vi "Dashboard Main.vi"() -> ()   [LabVIEW 2015]
uses:
  <vilib>/Utility/miscctls.llb/LVRowAndColumnTypeDef.ctl
  <vilib>/event_ctls.llb/eventvkey.ctl
  <vilib>/Rock Robotics/WPI/Dashboard/WPI_DashboardLogging Global.vi
  <vilib>/Rock Robotics/Network Tables/NT Read Numeric Array.vi
  <vilib>/Rock Robotics/Network Tables/NT Read Boolean.vi
  <vilib>/Rock Robotics/Network Tables/NT Write Boolean.vi
  <vilib>/functionblocks/Edge Detection/One Shot Rising with Input/One Shot Rising with Input.vi
  <vilib>/Utility/config.llb/Write Key (String).vi
  <vilib>/Utility/config.llb/Write Key (I32).vi
  <vilib>/functionblocks/FB Core/FB Core.xnode
  <vilib>/Utility/config.llb/NI_LVConfig.lvlib
  <vilib>/functionblocks/NI_FunctionBlock Libraries.lvlib
panel:
  in  "TCP":refnum<k5>
  in  "Rec Mode":enum32{"Stop", "Record", "Playback"}(radio)
  in  "Vision":u16(ring) items=["Camera Off", "USB Camera SW", "USB Camera HW", "IP Camera"]
  out "Camera IP":string
  out "Image Message":string="Timeout in Camera Communications"
  in  "Dashboard Tab":T1(tab)
  in  "Select Auto":string(combo)
  out "NT Connection":bool
  in  "Camera Settings":T2={"Frame Rate"=30, "Compression"=30, "Size"=1} {"Frame Rate" scale=1.0..30.0; "Size" items=["640x480", "320x240", "160x120"]}
  out "MotorChart R":cluster{"Numeric":dbl, "Numeric":dbl}(graph)
  out "MotorChart L":T3(graph)
  out "MotorSliders R":cluster{"MotorSlide1":dbl, "MotorSlide2":dbl} {"MotorSlide2" scale=-1.0..1.0 scale format="%#_2e"; "MotorSlide1" scale=-1.0..1.0 scale format="%#_2e"}
  out "MotorSliders L":T4 {"MotorSlide4 2" scale=0.0..14.0 scale format="%#_2e"; "MotorSlide2" scale=-1.0..1.0 scale format="%#_2e"; "MotorSlide1" scale=-1.0..1.0 scale format="%#_2e"}
  out "Gyro":dbl(knob) scale=0.0..360.0
  out "JS1 Z":dbl(slide) scale=-1.0..1.0 scale format="%#_2e"
  out "JS1 Graph":cluster{"X":dbl, "Y":dbl}[](graph)
  out "JS1 Buttons":T5
  out "JS2 Z":dbl(slide) scale=-1.0..1.0 scale format="%#_2e"
  out "JS2 Graph":cluster{"X":dbl, "Y":dbl}[](graph)
  out "JS2 Buttons":T5
  out "Mode":T6(ring)=enum."Auto Disabled"
  in  "DB Camera Config":bool
  out "fps":dbl format="%#.1g"
  out "Mbps":dbl format="%#.1g"
  out "Mbps LED":bool
  out "Image Out":T7(plugin-control)
  out "Drawing Box":bool
  in  "Auto Mode":enum16{"No Auto", "Simple Auto", "Shoot Auto"}(ring)
  in  "Push Camera Values":bool
  in  "Sat Min":dbl
  in  "Sat Max":dbl
  in  "Val Min":dbl
  in  "Val Max":dbl
  in  "Hue Min":dbl
  in  "Hue Max":dbl
  in  "Camera calibration":bool
  out "SHOOTER FAULT":bool
  out "Mode":string
  out "Shooter":dbl(slide) scale=0.0..80000.0
  out "Tilt":dbl(slide) scale=0.0..750.0
  out "Elevation":dbl(slide) scale=0.0..45000.0
  out "ELEVATOR FAULT":bool
  out "TILT FAULT":bool
  in  "Test Slider":dbl(slide) scale=0.0..100.0 scale format="%#_3g"
  in  "On/Off":bool caption="Solenoid"
  in  "Test Name":u16(ring) items=["Select the test to run..."]
  in  "Test Tree":string(tree)
  in  "Motor":cluster{"Value":dbl, "Enable":bool} {"Value" scale=-1.0..1.0 scale format="%#_3g"}
  out "Progress":T8 {"Test Progress" scale=0.0..100.0}
  in  "Rev/Fwd":cluster{"Forward":bool, "Reverse":bool}
  in  "Test Ring":u16(ring) items=["Monochrome", "Color"]
  out "Cmd Status":string
  in  "Execute Command":bool
  in  "Command Params":string[][](table)
  in  "Command Selection":i32(listbox)
  in  "CheckList":i32(listbox)
  out "Tree":string(tree)
  out "Camera Image":T7(plugin-control)
  out "Background":bool
  # "Left"
  # "Front"
  # "Right"
  # "Battery"
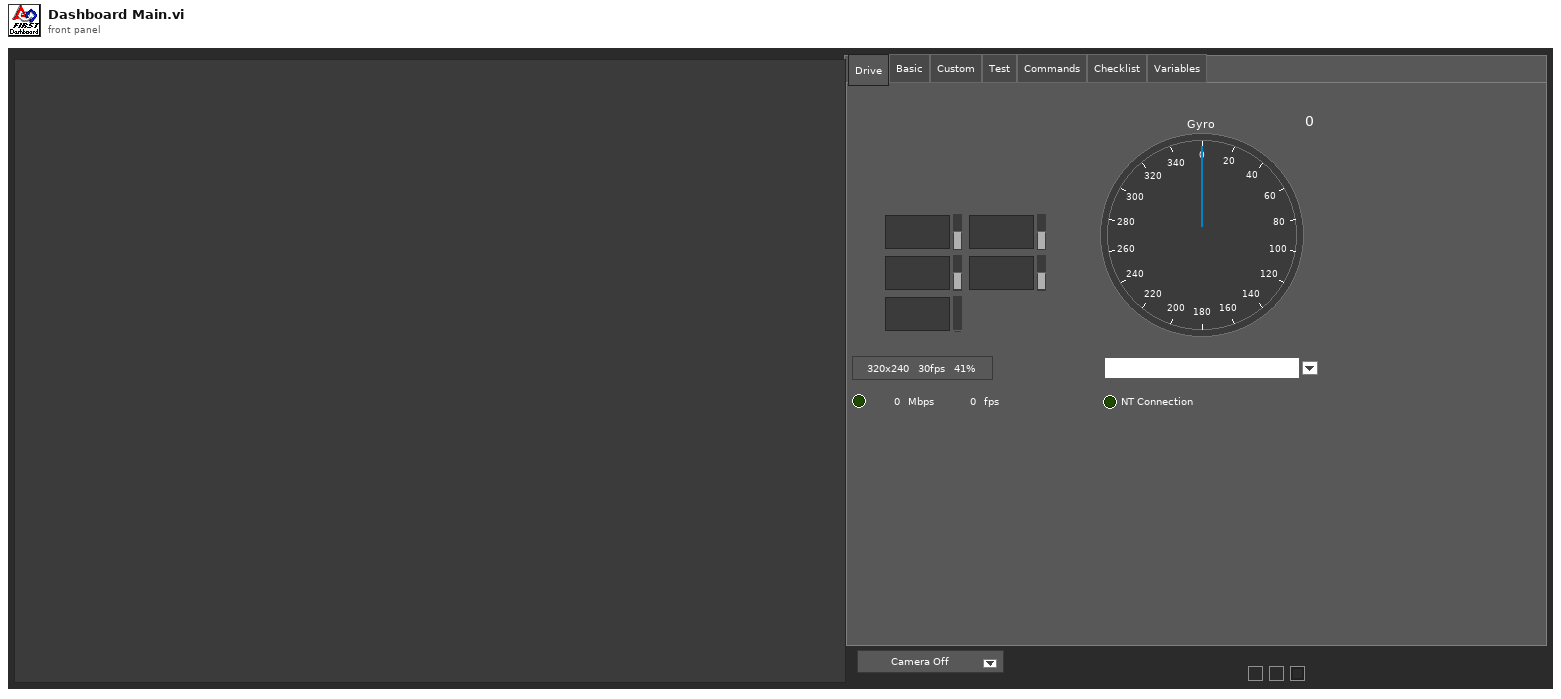
[diagram p1: front panel]
types:
  T1 = enum32{"Drive", "Basic", "Custom", "Test", "Commands", "Checklist", "Variables"}
  T2 = cluster{"Frame Rate":i32, "Compression":i32, "Size":u16}
  T3 = cluster{"Numeric":dbl, "Numeric":dbl, "Battery V":dbl}
  T4 = cluster{"MotorSlide1":dbl, "MotorSlide2":dbl, "MotorSlide4 2":dbl}
  T5 = cluster{bool, bool, bool, bool, bool, bool, bool, bool, bool, bool, bool, bool}
  T6 = enum8{"Tele-Op Disabled", "Tele-Op Enabled", "Auto Disabled", "Auto Enabled", "Test Disabled", "Test Enabled", "Disconnected", "No Code", "E-Stop"}
  T7 = typedef "IMAQ Image.ctl" = refnum<image>
  T8 = cluster{"Test Progress":u8, "Test Progress Text":string}
  T9 = cluster{"IDs":cluster{"RPC field ID":u16, "Unique ID":u16}, "String":string}
  T10 = enum32{"Drive", "Basic", "Custom", "Test", "Checklist", "Variables"}
  T11 = typedef "Image Type" = u32
  T12 = cluster{"Camera Image":refnum<vi>, "Dashboard Tab":refnum<vi>, "Background":refnum<vi>, "Vision":refnum<vi>, "Rec Mode":refnum<vi>, "Test Slider":refnum<vi>, "On/Off ":refnum<vi>, "Test Ring":refnum<vi>, "Rev/Fwd":refnum<vi>, "Test Name":refnum<vi>, "Motor":refnum<vi>, "Progress":refnum<vi>, "CheckList":refnum<vi>, "Tree":refnum<vi>, "Test Tree":refnum<vi>, "Command Params":refnum<vi>, "Command Selection":refnum<vi>, "Execute Command":refnum<vi>, "Cmd Status":refnum<vi>}
  T13 = cluster{"Error Strings":string, "Disable Counts":cluster{u16, u16}, "Rail Faults":cluster{u16, u16, u16}, "Robot IP":string, "DB Mode":u8, "Event Info":cluster{"Name":string, "Type":u8, "Number":u16, "Replay":u8}, "Camera Addr":string}
  T14 = cluster{"Storage":cluster{"Disk Free":u64, "RAM Block":u32, "RAM free":u32}, "CPU Utilization":cluster{"CPU % ISR":sgl, "CPU % Time Crit":sgl, "CPU % Timed Str":sgl, "CPU % High":sgl, "CPU % Above":sgl, "CPU % Normal":sgl, "CPU % Low":sgl}, "CAN":cluster{"% Bus Utilization":sgl, "Bus Off Cnt":u32, "TX_FIFO Full Cnt":u32, "Receive Error Cnt":u8, "Transmit Error Cnt":u8}, "HID":cluster{"HID Outputs":u32, "Rumble Low":u16, "Rumble High":u16}[]}
  T15 = cluster{"Status bits":cluster{"Test Mode":bool, "Autonomous":bool, "Enabled":bool, "Code Start":bool, "Brownout":bool, "Reserved 2":bool, "Reserved 3":bool, "E-Stop":bool}, "Code Trace":cluster{"Disabled":bool, "TeleOp":bool, "Auto":bool, "Test":bool}, "Controller Type":enum16{"unknown", "cRIO", "roboRio"}, "Code?":enum16{"unknown", "noCode", "code"}, "Battery V":dbl}
  T16 = cluster{"Control Bits":cluster{"TestMode":bool, "Autonomous":bool, "Enabled":bool, "FMS Present":bool, bool, bool, bool, "E-Stop":bool}, "Team Station ":u8, "Countdown":sgl, "Joystick Values":cluster{"Axes":dbl[], "Buttons":bool[], "POVs":i16[]}[]}
  T17 = cluster{"Axes":dbl[], "Buttons":bool[], "POVs":i16[]}[]
  T18 = cluster{"Axes":dbl[], "Buttons":bool[], "POVs":i16[]}
  T19 = cluster{"Buttons[0]":bool, "Buttons[1]":bool, "Buttons[2]":bool, "Buttons[3]":bool, "Buttons[4]":bool, "Buttons[5]":bool, "Buttons[6]":bool, "Buttons[7]":bool, "Buttons[8]":bool, "Buttons[9]":bool, "Buttons[10]":bool, "Buttons[11]":bool}
  T20 = typedef "NI_LVConfig.lvlib/Config Data RefNum.ctl" = refnum<k1>
  T21 = cluster{"Operation":enum16{"Update", "Clear"}, "Color Box":u32}[]
  T22 = typedef "eventvkey.ctl" = enum16{"ASCII", "Enter", "Return", "Shift", "Ctrl", "Alt", "Cmd", "Opt", "Caps", "NumLock", "Clear", "Break", "Up", "Down", "Left", "Right", "Insert", "Delete", "Home", "End", "PageUp", "PageDown", "Escape", "Help", "Pause", "ScrollLock", "F1", "F2", "F3", "F4", "F5", "F6", "F7", "F8", "F9", "F10", "F11", "F12", "F13", "F14", "F15", "F16", "F17", "F18", "F19", "F20", "F21", "F22", "F23", "F24", "Play", "VolumeUp", "VolumeDown", "Mute", "Two Byte Char"}
  T23 = cluster{"Image Size":bool, "Image Type":bool, "Pixel Value":bool, "ROI Information":bool, "Zoom Factor":bool}
  T24 = enum8{"Enabled", "Disabled", "Disabled and Grayed Out"}
  T25 = cluster{"Operation":enum16{"Update", "Clear"}, "Color Box":u32}
  T26 = typedef "LVRowAndColumnTypeDef.ctl" = cluster{"Row":i32, "Column":i32}
  T27 = cluster{"Shift":bool, "Ctrl":bool, "Alt":bool, "Cmd":bool, "Opt":bool}
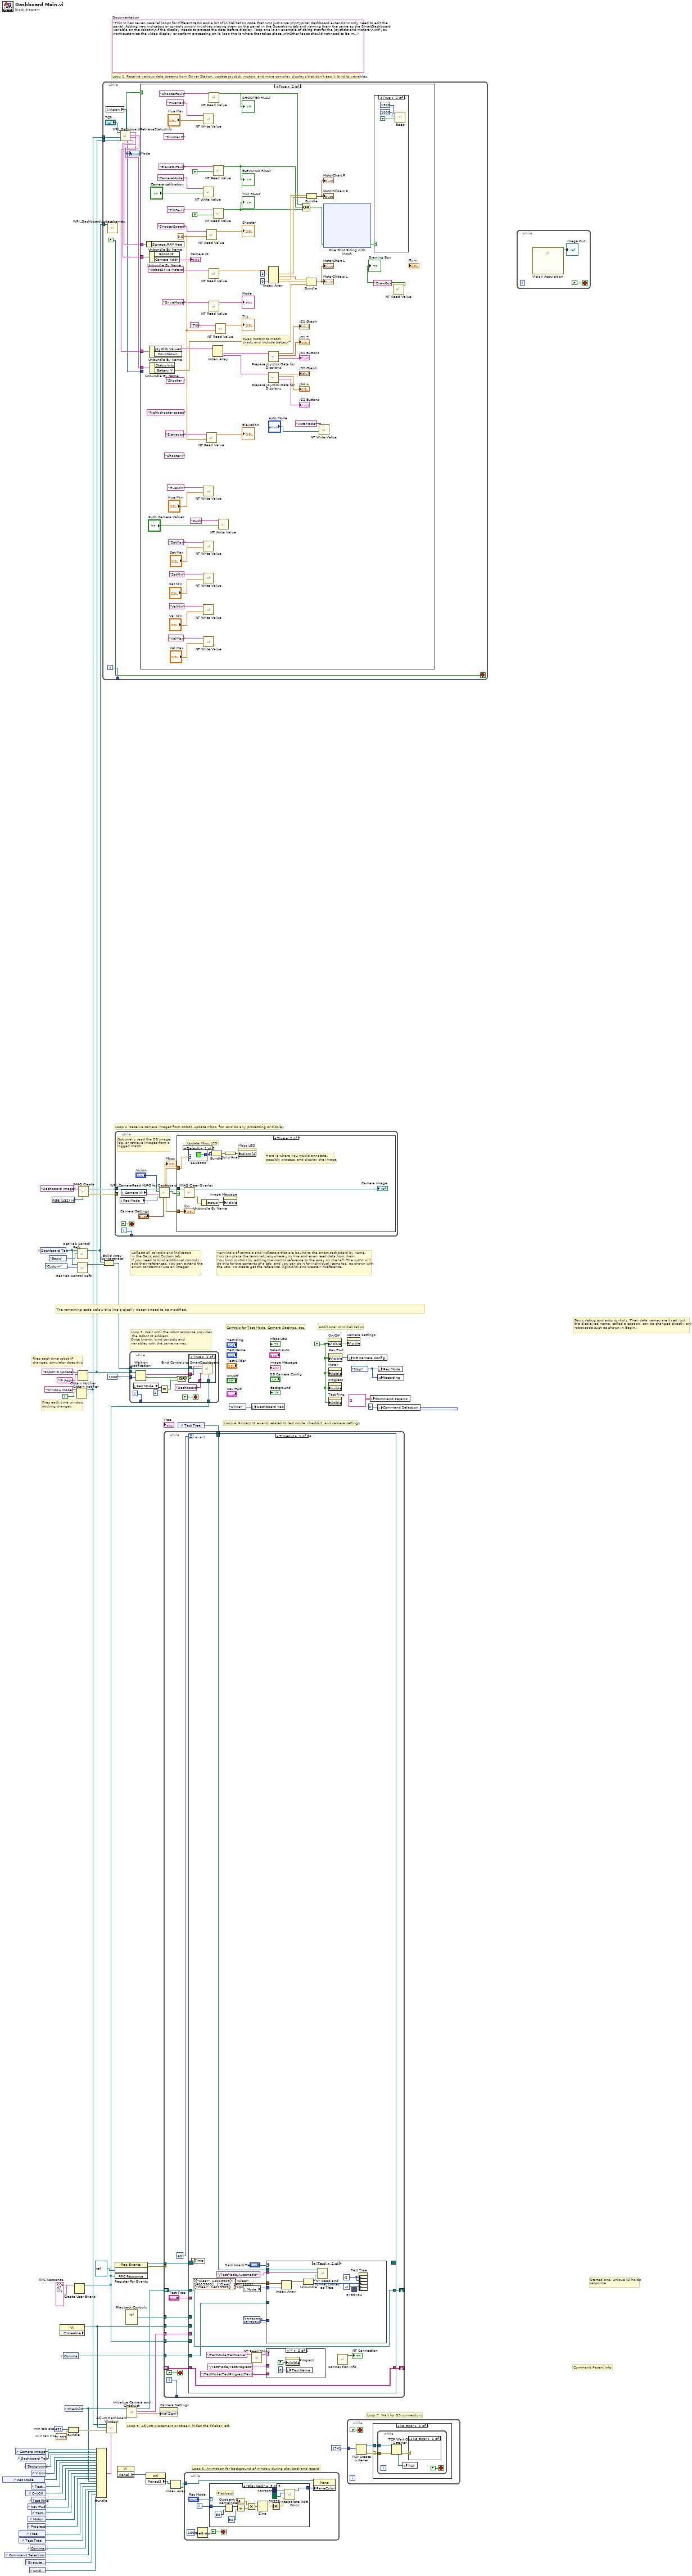
[diagram p0: block diagram]
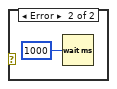
[diagram p2: hidden frame]
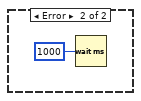
[diagram p3: hidden frame]
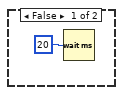
[diagram p4: hidden frame]
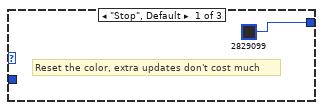
[diagram p6: hidden frame]
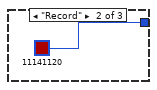
[diagram p7: hidden frame]
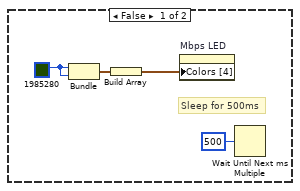
[diagram p9: hidden frame]
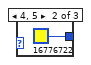
[diagram p10: hidden frame]
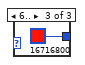
[diagram p11: hidden frame]
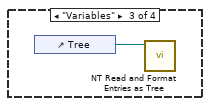
[diagram p13: hidden frame]
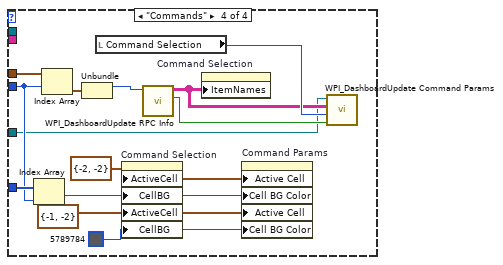
[diagram p14: hidden frame]
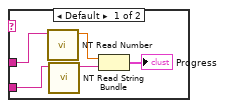
[diagram p15: hidden frame]
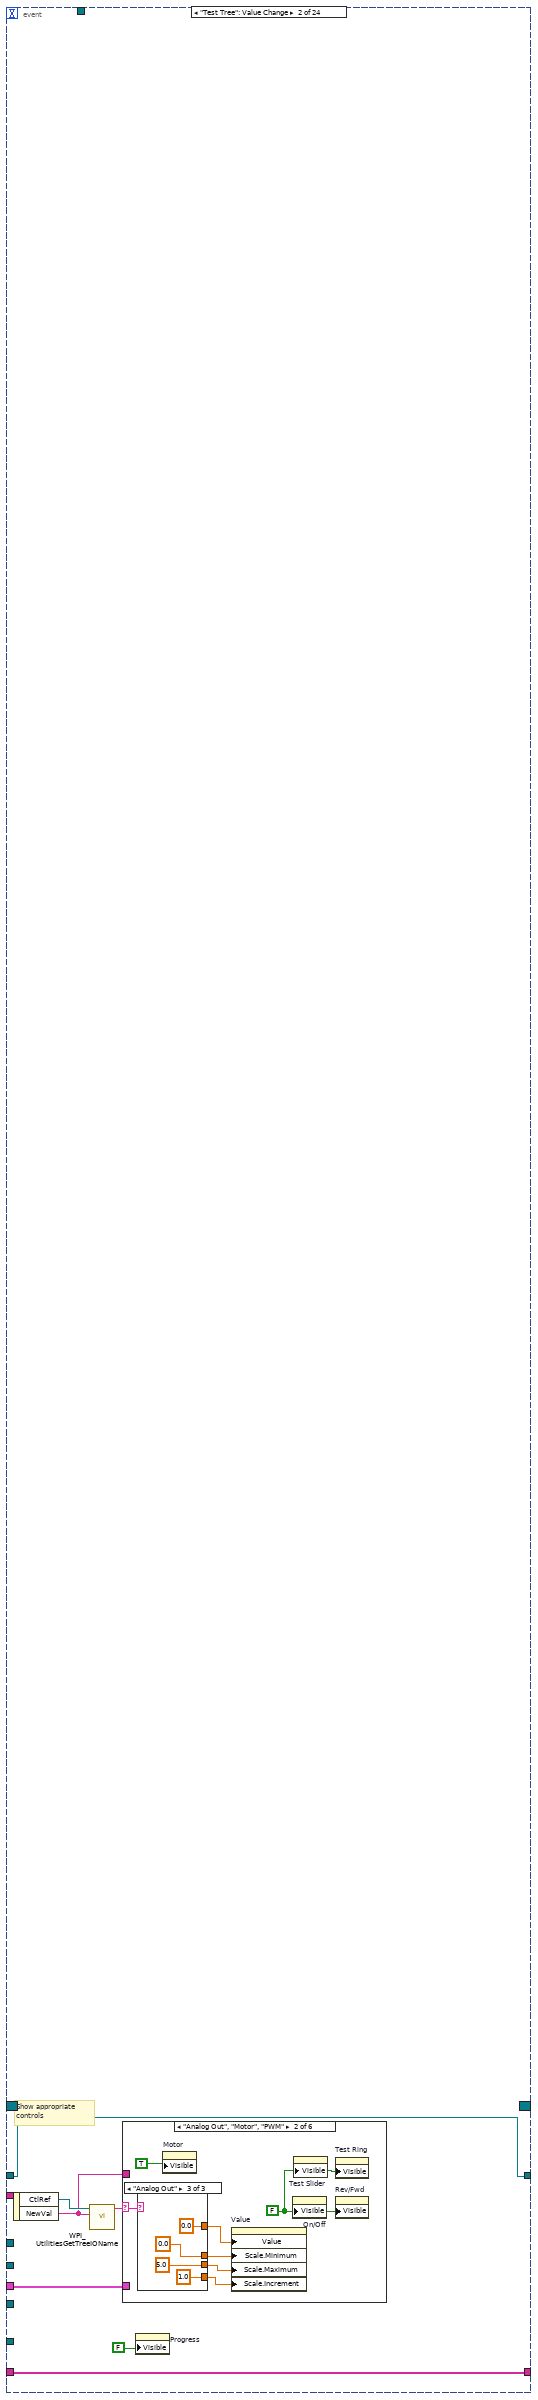
[diagram p16: hidden frame]
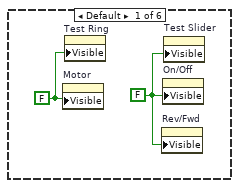
[diagram p17: hidden frame]
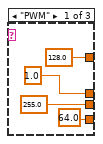
[diagram p18: hidden frame]
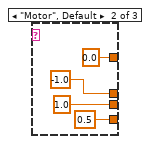
[diagram p19: hidden frame]
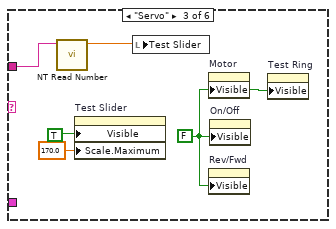
[diagram p20: hidden frame]
diagram:
  w7 = T9 {"IDs"={"RPC field ID"=0, "Unique ID"=0}, "String"=""}  # RPC Response
  w33 = 491  # min tab size
  w32 = 1.333  # min tab size
  w41 = enum32{"Stop", "Record", "Playback"}."Stop" ("Rec Mode")
  w15 = FALSE ("Visible")
  (unwired) "This VI has seven parallel loops for different tasks and a bit of initialization code that runs just once.\n\nTypical dashboard extensions only need to edit the panel. Adding new indicators or controls simply involves placing them on the panel in the Operations tab and naming them the same as the SmartDashboard variable on the robot\n\nIf the display needs to process the data before display, loop one is an example of doing that for the joysticks and motors.\n\nIf you want customize the video display or perform processing on it, loop two is where that takes place.\n\nOther loops should not need to be modified. They are pretty standard, and document the task they perform."  # Documentation
  w61 = T11 4 items=["Grayscale (U8)", "Grayscale (I16)", "Grayscale (SGL)", "Complex (CSG)", "RGB (U32)", "HSL (U32)", "RGB (U64)"] ("Image Type")
  # "Command Param Info"
  # "Started one, Unique ID holds\nresponse"
  # "Loop 7. Wait for DS connections"
  # "Basic debug and auto controls: Their data names are fixed, but\nthe displayed name, called a caption, can be changed directly or in\nrobot code such as shown in Begin."
  # "Controls for Test Mode, Camera Settings, etc."
  # "Additional UI Initialization"
  # "Loop 6. Animation for background of window during playback and record"
  # "Fires each time robot IP\nchanges, simulator does this"
  # "Fires each time window\ndocking changes."
  # "Collects all controls and indicators\nin the Basic and Custom tab.\nIf you need to bind additional controls,\nadd their references. You can extend the\nenum constant or use an integer."
  # "The remaining code below this line typically doesn't need to be modified."
  # "Loop 4. Process UI events related to test mode, checklist, and camera settings"
  # "Terminals of controls and indicators that are bound to the smart dashboard by name.\nYou can place the terminals anywhere you like and even read data from them.\nYou bind controls by adding the control reference to the array on the left. The subVI will\ndo this for the contents of a tab, and you can do it for individual items too, as shown with\nthe LED. To create get the reference, right-click and Create>>Reference."
  # "Loop 3. Wait until the robot response provides\n the Robot IP address.\nOnce known, bind controls and\nvariables with the same names."
  # "Loop 5. Adjusts placement onscreen, hides the titlebar, etc."
  # "Loop 1. Receive various data streams from Driver Station, update joystick, motors, and more complex displays that don't easily bind to variables."
  # "Loop 2. Receive camera images from Robot, update Mbps, fps, and do any processing or display"
  n1 = control-ref of="Rec Mode"() -> (w21:refnum<vi>)
  n2 = control-ref of="Command Selection"() -> (w6:refnum<vi>)
  n3 = control-ref of="Camera Image"() -> (w36:refnum<vi>)
  n4 = control-ref of="Tree"() -> (w25:refnum<vi>)
  n5 = control-ref of="Test Tree"() -> (w24:refnum<vi>)
  n6 = control-ref of="Dashboard Tab"() -> (w35:refnum<vi>)
  n7 = control-ref of="Execute Command"() -> (w8:refnum<vi>)
  n8 = control-ref of="Background"() -> (w30:refnum<vi>)
  n9 = control-ref of="On/Off"() -> (w19:refnum<vi>)
  n10 = control-ref of="Progress"() -> (w16:refnum<vi>)
  n11 = control-ref of="Rev/Fwd"() -> (w17:refnum<vi>)
  n12 = control-ref of="Motor"() -> (w22:refnum<vi>)
  n13 = control-ref of="Cmd Status"() -> (w2:refnum<vi>)
  n14 = control-ref of="Command Params"() -> (w9:refnum<vi>)
  n15 = control-ref of="Test Slider"() -> (w20:refnum<vi>)
  n16 = control-ref of="Vision"() -> (w34:refnum<vi>)
  n17 = control-ref of="Test Ring"() -> (w18:refnum<vi>)
  n18 = control-ref of="Test Name"() -> (w23:refnum<vi>)
  n19 = control-ref of="Dashboard Tab"() -> (w39:refnum<vi>)
  n20 = property class="VI" props=["Front Panel.Closeable"]() -> (reference out=w40:refnum<vi>)  [unwired: 2 in, 2 out]
  n21 = control-ref of="Command Params"() -> (w1:refnum<vi>)
  n22 = control-ref of="CheckList"() -> (w26:refnum<vi>)
  n23 = Bundle("min tab size"=w33, "min tab size"=w32) -> (w31:cluster{"min tab size":i32, "min tab size":dbl})  [unwired: 1 in]
  n24 = Create User Event(user event datatype=w7) -> (user event=w3:refnum<user-event>)  [unwired: 1 in, 1 out]
  n25 = Obtain Notifier(name (unnamed)="Window Mode", notification data type=TRUE) -> (notifier out=w12:refnum<notifier>)  [unwired: 2 in, 2 out]
  n26 = call <vilib>:"Get Tab Control Refs.vi"("Page Index"=T10."Basic" ("Dashboard Tab"), "TabControl in"=w39) -> ("ControlsOnPage"=w13:refnum<vi>[])  [unwired: 9 in]
  n27 = call <vilib>:"Get Tab Control Refs.vi"("Page Index"=T10."Custom" ("Dashboard Tab"), "TabControl in"=w39) -> ("ControlsOnPage"=w38:refnum<vi>[])  [unwired: 9 in]
  n28 = Obtain Notifier(name (unnamed)="Robot IP Update", notification data type="IP Addr" ("name (unnamed)")) -> (notifier out=w14:refnum<notifier>)  [unwired: 2 in, 2 out]
  n29 = call "IMAQ Create"("Image Name"="Dashboard Image", "Image Type"=w61) -> ("New Image"=w59:T7, "error out"=w58:errorcluster)  [unwired: 2 in, 1 out]
  n30 = Bundle("Camera Image"=w36, "Dashboard Tab"=w35, "Background"=w30, "Vision"=w34, "Rec Mode"=w21, "Test Slider"=w20, "On/Off"=w19, "Test Ring"=w18, "Rev/Fwd"=w17, "Test Name"=w23, "Motor"=w22, "Progress"=w16, "CheckList"=w26, "Tree"=w25, "Test Tree"=w24, "Command Params"=w9, "Command Selection"=w6, "Execute Command"=w8, "Cmd Status"=w2) -> (w27:T12)  [unwired: 1 in]
  n31 = while {
    tunnel: [w73] -> _
    tunnel: w14 -> [w67]
    tunnel: w13 -> [w66]
    tunnel: w12 -> [w62]
    i -> [w73]
    stop <- FALSE stop-if-true
    n32 = local read "Vision"() -> (w64:u16)
    n33 = call <vilib>:"WPI_DashboardUpdateNames.vi"("Controls on Tab"=w66) -> ()  [unwired: 11 in]
    n34 = call <vilib>:"WPI_DashboardRetrieveStatusInfo.vi"("Vision"=w64, "Binding Refnum"=w67, "Window Mode Notifier"=w62, "TCP Cnx"="TCP") -> ("Power and Errors"=w68:T13, "Robot Metrics"=w71:T14, "Status Info"=w72:T15, "Control Info"=w69:T16, "Robot Mode"=w65:T6, "Process?"=w70:bool)  [unwired: 2 in]
    "Mode" <- w65
    n35 = case shown="True" w70 {
      tunnel: w72 -> [_ w139]
      tunnel: w71 -> [_ w138]
      tunnel: w69 -> [_ w137]
      tunnel: w68 -> [_ w136]
      tunnel: w65 -> [_ _]
      frame False {
        n36 = Wait (ms)(milliseconds to wait=u32 20) -> ()  [unwired: 1 out]
      }
      frame True {
        (unwired) "Shooter D" ("Name")
        (unwired) "Shooter I" ("Name")
        (unwired) "Shooter P" ("Name")
        (unwired) "Right shooter speed" ("Name")
        w105 = 0.0 ("Default Value")
        # "swap motors to match\ncharts and include battery"
        n37 = Unbundle By Name(w138) -> ()  [unwired: 1 out]
        n38 = Unbundle By Name(w137) -> ("Joystick Values"=w126:T17)  [unwired: 1 out]
        n39 = Unbundle By Name(w136) -> ("Camera Addr"=→"Camera IP":string)  [unwired: 1 out]
        n40 = Unbundle By Name(w139) -> ("Battery V"=w127:dbl)  [unwired: 1 out]
        n41 = call-poly <vilib>:"NT Write Value.vi"("Boolean"="Camera calibration", "Name"="CameraMode") -> ()  [unwired: 9 in, 1 out]
        n42 = call-poly <vilib>:"NT Write Value.vi"("Numeric"="Hue Max", "Name"="HueMax") -> ()  [unwired: 9 in, 1 out]
        n43 = call-poly <vilib>:"NT Write Value.vi"("Numeric"="Hue Min", "Name"="HueMin") -> ()  [unwired: 9 in, 1 out]
        n44 = call-poly <vilib>:"NT Write Value.vi"("Numeric"="Sat Max", "Name"="SatMax") -> ()  [unwired: 9 in, 1 out]
        n45 = call-poly <vilib>:"NT Write Value.vi"("Numeric"="Sat Min", "Name"="SatMin") -> ()  [unwired: 9 in, 1 out]
        n46 = call-poly <vilib>:"NT Write Value.vi"("Numeric"="Val Min", "Name"="ValMin") -> ()  [unwired: 9 in, 1 out]
        n47 = call-poly <vilib>:"NT Write Value.vi"("Numeric"="Val Max", "Name"="ValMax") -> ()  [unwired: 9 in, 1 out]
        n48 = call-poly <vilib>:"NT Read Value.vi"("Default Value"=w105, "Name"="ShooterSpeed") -> ("Numeric"=→"Shooter":dbl)  [unwired: 8 in, 1 out]
        n49 = call-poly <vilib>:"NT Read Value.vi"("Default Value"=w105, "Name"="Elevation") -> ("Numeric"=→"Elevation":dbl)  [unwired: 8 in, 1 out]
        n50 = call-poly <vilib>:"NT Read Value.vi"("Name"="ShooterFault") -> ("Boolean"=w100:bool)  [unwired: 9 in, 1 out]
        "SHOOTER FAULT" <- w100
        n51 = call-poly <vilib>:"NT Read Value.vi"("Name"="RobotDrive Motors") -> ("Numeric Array"=w115:dbl[])  [unwired: 9 in, 1 out]
        n52 = call-poly <vilib>:"NT Read Value.vi"("Name"="DriveMode") -> ("String"=→"Mode":string)  [unwired: 9 in, 1 out]
        n53 = Index Array(array=w126) -> (element #1=w125:T18, element #2=w120:T18)  [unwired: 2 in]
        n54 = call-poly <vilib>:"NT Read Value.vi"("Default Value"=FALSE, "Name"="ElevatorFault") -> ("Boolean"=w101:bool)  [unwired: 8 in, 1 out]
        "ELEVATOR FAULT" <- w101
        n55 = call-poly <vilib>:"NT Read Value.vi"("Default Value"=FALSE, "Name"="TiltFault") -> ("Boolean"=w99:bool)  [unwired: 8 in, 1 out]
        "TILT FAULT" <- w99
        n56 = call-poly <vilib>:"NT Read Value.vi"("Default Value"=w105, "Name"="Tilt") -> ("Numeric"=→"Tilt":dbl)  [unwired: 8 in, 1 out]
        n57 = call-poly <vilib>:"NT Write Value.vi"("Boolean"="Push Camera Values", "Name"="Push") -> ()  [unwired: 9 in, 1 out]
        n58 = Index Array(array=w115, index #1=1, index #4=0) -> (element #1=w131:dbl, element #2=w132:dbl, element #3=w130:dbl, element #4=w135:dbl)  [unwired: 2 in]
        n59 = call "Prepare Joystick Data for Displays.vi"("Joystick Values"=w125) -> ("Buttons"=→"JS1 Buttons":T19, "Z Axis"=→"JS1 Z":dbl, "Cartesian Data"=→"JS1 Graph":cluster{"X axis":dbl, "X axis":dbl}[])  [unwired: 8 in]
        n60 = call "Prepare Joystick Data for Displays.vi"("Joystick Values"=w120) -> ("Buttons"=→"JS2 Buttons":T19, "Z Axis"=→"JS2 Z":dbl, "Cartesian Data"=→"JS2 Graph":cluster{"X axis":dbl, "X axis":dbl}[])  [unwired: 8 in]
        n61 = Compound Arithmetic op=OR(w100, w101, w99) -> (w98:bool)
        n62 = Bundle("Numeric"=w132, "Numeric"=w135, "Battery V"=w127) -> (→"MotorChart L" →"MotorSliders L":T3)  [unwired: 1 in]
        n63 = Bundle("Numeric"=w130, "Numeric"=w131) -> (→"MotorChart R" →"MotorSliders R":cluster{"Numeric":dbl, "Numeric":dbl})  [unwired: 1 in]
        n64 = call-poly <vilib>:"NT Write Value.vi"("Numeric"="Auto Mode", "Name"="AutoMode") -> ()  [unwired: 9 in, 1 out]
        n65 = xnode "One Shot Rising with Input"("input"=w98) -> ("output"=w97:bool)  [unwired: 1 in, 1 out]
        n66 = case shown="True" w97 {
          frame False {
          }
          frame True {
            n67 = call <vilib>:"Beep.vi"("use system alert? (T)"=FALSE, "duration (msec)"=u32 1000, "frequency (Hz)"=u32 1500) -> ()  [unwired: 9 in]
          }
        }
        n68 = call-poly <vilib>:"NT Read Value.vi"("Name"="DrawBox") -> ("Boolean"=→"Drawing Box":bool)  [unwired: 9 in, 1 out]
      }
    }
  }
  n69 = Build Array (concatenate)(w13, w38) -> (w37:refnum<vi>[])
  n70 = call "Adjust Dashboard Window.vi"("Sizing Refnums"=w27, "Size Constraints"=w31, "VI"=w40, "WIn Mode"=w12) -> ()  [unwired: 8 in]
  n71 = while {
    tunnel: w59 -> [w189]
    tunnel: w58 -> [_]
    tunnel: [w190] -> _
    i -> [w190]
    stop <- FALSE stop-if-true
    # "Optionally read the DB image,\nlog, or retrieve images from a\nlogged match"
    n72 = local read "Rec Mode"() -> (w184:enum32{"Stop", "Record", "Playback"})
    n73 = local read "Camera IP"() -> (w182:string)
    n74 = call <vilib>:"WPI_CameraRead MJPG for Dashboard.vi"("Camera Settings"="Camera Settings", "Rec Mode"=w184, "Camera IP"=w182, "Camera Mode"="Vision", "Refnum in"=w189) -> ("Active"=w187:bool, "Refnum out"=w188:T7, "FPS"=w186:dbl, "Bandwidth (Mbps)"=w181:dbl)  [unwired: 3 in]
    "Mbps" <- w181
    n75 = case shown="True" w187 {
      tunnel: w188 -> [_ w199]
      tunnel: w181 -> [_ w198]
      tunnel: w186 -> [_ w196]
      frame False {
        w192 = u32 1985280 ("Color Box")
        # "Sleep for 500ms"
        n76 = Bundle("Color Box"=w192, "Color Box"=w192) -> (w194:cluster{"Color Box":u32, "Color Box":u32})  [unwired: 1 out]
        n77 = Build Array(w194) -> (w193:cluster{"Color Box":u32, "Color Box":u32}[])
        n78 = property on="Mbps LED" class="Bool (strict)"("Colors [4]"=w193) -> ()  [unwired: 2 in, 2 out]
        n79 = Wait Until Next ms Multiple(millisecond multiple=u32 500) -> ()  [unwired: 1 out]
      }
      frame True {
        # "Here is where you would annotate,\npossibly process, and display the image"
        # "Update Mbps LED"
        n80 = call "IMAQ Clear Overlay"("Image"=w199) -> ("error out"=w203:errorcluster, "Image Out"=→"Camera Image":T7)  [unwired: 2 in, 7 out]
        n81 = case shown="Default" w198 {
          tunnel: [u32 6618880 ("Color Box") u32 16776722 ("Color Box") u32 16716800 ("Color Box")] -> w200
          frame Default {
          }
          frame 4, 5 {
          }
          frame 6.. {
          }
        }
        n82 = Unbundle By Name(w203) -> ("status"=w204:bool)
        n83 = Bundle("Color Box"=w200, "Color Box"=w200) -> (w202:cluster{"Color Box":u32, "Color Box":u32})  [unwired: 1 out]
        n84 = property on="Image Message" class="Str"("Visible"=w204) -> ()  [unwired: 2 in, 2 out]
        n85 = Build Array(w202) -> (w201:cluster{"Color Box":u32, "Color Box":u32}[])
        n86 = property on="Mbps LED" class="Bool (strict)"("Colors [4]"=w201) -> ()  [unwired: 2 in, 2 out]
        "fps" <- w196
      }
    }
  }
  n87 = register-events(refnum<vi> refnum, w3) -> (reference out=w45:refnum<event-registration>, error out=w44:errorcluster)  [unwired: 2 in]
  n88 = property class="VI"() -> ("Panel"=w48:refnum<vi>)  [unwired: 2 in, 2 out]
  n89 = vi-ref "Playback Controls.vi"() -> (w46:refnum<vi>)
  n90 = call "Initialize Camera and CheckList.vi"("ListBox in"=w26) -> ("Cluster"=w52:cluster{"value":i32, "value":i32, "index":i32}, "Array"=w53:cluster{string[]}[], "File Refnum"=w51:T20)  [unwired: 8 in]
  n91 = while {
    tunnel: w37 -> [w220]
    tunnel: w14 -> [w218]
    tunnel: [w216] -> _
    tunnel: u32 1000 ("milliseconds to wait") -> [w215]
    tunnel: w3 -> [w208]
    i -> [w216]
    stop <- FALSE stop-if-true
    n92 = local read "Rec Mode"() -> (w211:enum32{"Stop", "Record", "Playback"})
    n93 = Wait on Notification(notifier=w218, timeout in ms (-1)=w215) -> (notification=w217:string, timed out?=w213:bool)  [unwired: 2 in, 2 out]
    n94 = Equal?(x=w211, y=u16 2 ("Rec Mode")) -> (x = y?=w212:bool)
    n95 = Compound Arithmetic op=OR(invert w213, w212) -> (w214:bool)
    n96 = case shown="True" w214 {
      tunnel: w220 -> [_ w224]
      tunnel: w217 -> [_ w223]
      tunnel: "Dashboard" -> [_ w222]
      tunnel: w208 -> [_ w221]
      frame False {
      }
      frame True {
        n97 = call <vilib>:"Bind Controls to SmartDashboard.vi"("RPC ref"=w221, "Client Name"=w222, "Bound Control Refs"=w224, "Server IP Address"=w223) -> ()  [unwired: 8 in]
      }
    }
  }
  n98 = property class="Pnl"(reference=w48) -> ("Panes[]"=w49:refnum<vi>[])  [unwired: 1 in, 2 out]
  n99 = property on="Camera Settings" class="Clust (strict)"("Val(Sgnl)"=w52) -> ()  [unwired: 2 in, 2 out]
  n100 = Index Array(array=w49) -> (element=w47:refnum<vi>)  [unwired: 1 in]
  n101 = control-ref of="Test Tree"() -> (w50:refnum<vi>)
  n102 = while {
    tunnel: w53 -> [w236]
    shift-right: [w235] -> _
    shift-left: w51 -> [w234]
    tunnel: [w233] -> _
    tunnel: w50 -> [w232]
    tunnel: w46 -> [w231]
    tunnel: w45 -> [w230]
    tunnel: w44 -> [_]
    tunnel: w40 -> [w229]
    tunnel: w3 -> [w228]
    tunnel: w1 -> [w227]
    shift-right: [w226] -> _
    shift-left: _ -> [w225]
    i -> [w233]
    stop <- FALSE stop-if-true
    n103 = event shown="[0] Timeout" {
      selector: w230 -> [_ _ _ _ _ _ _ _ _ _ _ _ _ _ _ _ _ _ _ _ _ _ _ _]
      dyn-events: [_ _ _ _ _ _ _ _ _ _ _ _ _ _ _ _ _ _ w545 _ _ _ _ _] -> _
      timeout: u32 60 ("milliseconds to wait") -> [_ _ _ _ _ _ _ _ _ _ _ _ _ _ _ _ _ _ _ _ _ _ _ _]
      tunnel: w232 -> [w249 _ _ _ _ _ _ _ _ _ _ _ _ _ _ _ _ _ _ _ _ _ _ _]
      tunnel: "Test Tree" -> [_ _ _ _ _ _ _ _ _ _ _ _ _ w508 w517 w520 w525 w534 _ _ _ _ _ _]
      tunnel: w236 -> [_ w287 _ _ _ _ _ _ _ _ _ w470 w501 _ _ _ _ _ _ _ _ _ _ _]
      tunnel: [w246 w286 w390 w396 w406 w410 w416 w428 w436 w442 w455 w469 w494 w507 w515 w519 w524 w533 w547 w563 w565 w573 w584 w589] -> w235
      tunnel: w234 -> [w246 w286 w390 w396 w406 w410 w416 w428 w436 w442 w455 w468 w494 w507 w515 w519 w524 w533 w547 w563 w565 w573 w584 w589]
      tunnel: w231 -> [_ _ _ _ _ _ _ _ _ _ _ _ _ _ _ _ _ _ w548 _ w568 _ _ _]
      tunnel: w229 -> [_ _ _ _ _ _ _ _ _ _ _ _ _ _ _ _ _ _ w543 _ _ _ _ _]
      tunnel: w228 -> [_ _ _ _ _ _ _ _ _ _ _ _ _ _ _ _ _ _ w539 _ _ _ _ _]
      tunnel: w227 -> [w241 _ _ _ _ _ w414 _ _ _ _ _ _ _ _ _ _ _ _ _ _ _ _ _]
      tunnel: [w240 w285 w389 w395 w405 w411 w412 w422 w433 w441 w454 w467 w493 w506 w514 w518 w523 w532 w538 w561 w564 w569 w577 w590] -> w226
      tunnel: w225 -> [w240 w285 w389 w395 w405 w411 w412 _ _ w441 w454 w467 w493 w506 w514 w518 w523 w532 w538 w561 w564 w569 w577 w590]
      event Timeout {
        n104 = event-data() -> ()  [unwired: 1 in, 1 out]
        n105 = local read "Mode"() -> (w243:T6)
        n106 = call <vilib>:"NT Read String.vi"("Name"="/TestMode/TestName") -> ("String"=w252:string)  [unwired: 9 in, 1 out]
        n107 = case shown="\"Test\"" "Dashboard Tab" {
          tunnel: w249 -> [_ w263 _ _]
          tunnel: "/TestMode/Automatic/" ("Name Pattern") -> [_ w262 _ _]
          tunnel: T21 [{"Operation"=enum."Clear", "Color Box"=14013909}, {"Operation"=enum."Clear", "Color Box"=14013909}, {"Operation"=enum."Clear", "Color Box"=14013909}, {"Operation"=enum."Clear", "Color Box"=14013909}, {"Operation"=enum."Update", "Color Box"=14013909}, {"Operation"=enum."Update", "Color Box"=16777215}, {"Operation"=enum."Clear", "Color Box"=14013909}, {"Operation"=enum."Clear", "Color Box"=14013909}, {"Operation"=enum."Clear", "Color Box"=14013909}] -> [_ w255 _ w272]
          tunnel: w243 -> [_ w254 _ w271]
          tunnel: u32[] [15790320, 15790320, 15790320, 15790320, 16777215, 16777215, 15790320, 15790320, 15790320] -> [_ _ _ w277]
          tunnel: w241 -> [_ _ _ w265]
          frame "Custom", Default {
          }
          frame "Test" {
            w261 = -2 ("Active Item:Row Number")
            n108 = Index Array(array=w255, index=w254) -> (element=w256:T25)
            n109 = Unbundle(w256) -> ("Operation"=w257:enum16{"Update", "Clear"}, "Color Box"=w258:u32)
            n110 = call <vilib>:"NT Read and Format Entries as Tree.vi"("Operation"=w257, "Name Pattern"=w262, "Tree Refnum"=w263) -> ()  [unwired: 7 in, 2 out]
            n111 = property on="Test Tree" class="Tree (strict)"("Active Item Row Number"=w261, "ActiveColNum"=w261, "CellBG"=w258, "Active Item Row Number"=-1 ("Active Item:Row Number"), "CellBG"=u32 5789784 ("Color Box")) -> ()  [unwired: 2 in, 2 out]
          }
          frame "Variables" {
            n112 = control-ref of="Tree"() -> (w264:refnum<vi>)
            n113 = call <vilib>:"NT Read and Format Entries as Tree.vi"("Tree Refnum"=w264) -> ()  [unwired: 9 in, 2 out]
          }
          frame "Commands" {
            w273 = u32 5789784 ("Color Box")
            w274 = T26 {"Row"=-1, "Column"=-2} ("Active Cell:Active Cell")
            w276 = T26 {"Row"=-2, "Column"=-2} ("Active Cell:Active Cell")
            n114 = Index Array(array=w277, index=w271) -> (element=w275:u32)
            n115 = Index Array(array=w272, index=w271) -> (element=w270:T25)
            n116 = Unbundle(w270) -> ("Operation"=w269:enum16{"Update", "Clear"})  [unwired: 1 out]
            n117 = local read "Command Selection"() -> (w268:i32)
            n118 = property on="Command Selection" class="MCListbox (strict)"("ActiveCell"=w276, "CellBG"=w275, "ActiveCell"=w274, "CellBG"=w273) -> ()  [unwired: 2 in, 2 out]
            n119 = call <vilib>:"WPI_DashboardUpdate RPC Info.vi"("Operation"=w269) -> ("update"=w267:bool, "commands"=w266:string[][])  [unwired: 9 in]
            n120 = property on="Command Selection" class="MCListbox (strict)"("ItemNames"=w266) -> ()  [unwired: 2 in, 2 out]
            n121 = property on="Command Params" class="Tbl (strict)"("Active Cell"=w276, "Cell BG Color"=w275, "Active Cell"=w274, "Cell BG Color"=w273) -> ()  [unwired: 2 in, 2 out]
            n122 = call <vilib>:"WPI_DashboardUpdate Command Params.vi"("Update"=w267, "NewVal"=w268, "Commands"=w266, "Param Tbl"=w265) -> ()  [unwired: 7 in, 1 out]
          }
        }
        n123 = case shown="\"\"" w252 {
          tunnel: "/TestMode/TestProgress" ("Name") -> [w279 _]
          tunnel: "/TestMode/TestProgressText" ("Name") -> [w278 _]
          frame Default {
            n124 = call <vilib>:"NT Read Number.vi"("Name"=w279) -> ("Numeric"=w280:dbl)  [unwired: 9 in, 1 out]
            n125 = call <vilib>:"NT Read String.vi"("Name"=w278) -> ("String"=w281:string)  [unwired: 9 in, 1 out]
            n126 = Bundle("Numeric"=w280, "String"=w281) -> (→"Progress":cluster{"Numeric":dbl, "String":string})  [unwired: 1 in]
          }
          frame "" {
            n127 = property on="Progress" class="Clust (strict)"("Visible"=FALSE) -> ()  [unwired: 2 in, 2 out]
            n128 = local write "Test Name"(u16 0) -> ()
          }
        }
        n129 = call <vilib>:"Connextion Info.vi"() -> ("Connected"=→"NT Connection":bool)  [unwired: 10 in, 1 out]
      }
      event "Test Tree": Value Change {
        # "Show appropriate\ncontrols"
        n130 = event-data() -> ("CtlRef"=w290:refnum<vi>, "NewVal"=w288:string)  [unwired: 1 in]
        n131 = call <vilib>:"WPI_UtilitiesGetTreeIOName.vi"("NewVal"=w288, "TreeControl in"=w290) -> ("I/O Name"=w291:string)  [unwired: 9 in]
        n132 = case shown="\"Analog Out\", \"Motor\", \"PWM\"" w291 {
          selector: w291 -> [_ w298 _ w320 w329 _]
          tunnel: w288 -> [_ _ w317 w319 _ w336]
          tunnel: w287 -> [_ _ _ _ _ w335]
          frame Default {
            w293 = FALSE ("Visible")
            w292 = FALSE ("Visible")
            n133 = property on="Motor" class="Clust (strict)"("Visible"=w292) -> ()  [unwired: 2 in, 2 out]
            n134 = property on="Test Ring" class="Ring (strict)"("Visible"=w292) -> ()  [unwired: 2 in, 2 out]
            n135 = property on="Rev/Fwd" class="Clust (strict)"("Visible"=w293) -> ()  [unwired: 2 in, 2 out]
            n136 = property on="On/Off" class="Bool (strict)"("Visible"=w293) -> ()  [unwired: 2 in, 2 out]
            n137 = property on="Test Slider" class="Slide (strict)"("Visible"=w293) -> ()  [unwired: 2 in, 2 out]
          }
          frame "Analog Out", "Motor", "PWM" {
            w299 = FALSE ("Visible")
            n138 = case shown="\"Analog Out\"" w298 {
              tunnel: [1.0 ("Value") -1.0 ("Value") 0.0 ("Value")] -> w297
              tunnel: [255.0 ("Value") 1.0 ("Value") 5.0 ("Value")] -> w296
              tunnel: [128.0 ("Value") 0.0 ("Value") 0.0 ("Value")] -> w295
              tunnel: [64.0 ("Value") 0.5 ("Value") 1.0 ("Value")] -> w294
              frame "PWM" {
              }
              frame "Motor", Default {
              }
              frame "Analog Out" {
              }
            }
            n139 = property on="Motor" class="Clust (strict)"("Visible"=TRUE) -> ()  [unwired: 2 in, 2 out]
            n140 = property on="Value" class="Slide (strict)"("Value"=w295, "Scale.Minimum"=w297, "Scale.Maximum"=w296, "Scale.Increment"=w294) -> ()  [unwired: 2 in, 2 out]
            n141 = property on="On/Off" class="Bool (strict)"("Visible"=w299) -> ()  [unwired: 2 in, 2 out]
            n142 = property on="Test Slider" class="Slide (strict)"("Visible"=w299) -> ()  [unwired: 2 in, 2 out]
            n143 = property on="Test Ring" class="Ring (strict)"("Visible"=w299) -> ()  [unwired: 2 in, 2 out]
            n144 = property on="Rev/Fwd" class="Clust (strict)"("Visible"=w299) -> ()  [unwired: 2 in, 2 out]
          }
          frame "Servo" {
            w315 = FALSE ("Visible")
            n145 = call <vilib>:"NT Read Number.vi"("Name"=w317) -> ("Numeric"=w316:dbl)  [unwired: 9 in, 1 out]
            n146 = property on="Test Slider" class="Slide (strict)"("Visible"=TRUE, "Scale.Maximum"=170.0 ("Scale.Range:Maximum")) -> ()  [unwired: 2 in, 2 out]
            n147 = local write "Test Slider"(w316) -> ()
            n148 = property on="Motor" class="Clust (strict)"("Visible"=w315) -> ()  [unwired: 2 in, 2 out]
            n149 = property on="Rev/Fwd" class="Clust (strict)"("Visible"=w315) -> ()  [unwired: 2 in, 2 out]
            n150 = property on="On/Off" class="Bool (strict)"("Visible"=w315) -> ()  [unwired: 2 in, 2 out]
            n151 = property on="Test Ring" class="Ring (strict)"("Visible"=w315) -> ()  [unwired: 2 in, 2 out]
          }
          frame "Relay", "Solenoid" {
            w318 = FALSE ("Visible")
            n152 = property on="Motor" class="Clust (strict)"("Visible"=w318) -> ()  [unwired: 2 in, 2 out]
            n153 = property on="Test Slider" class="Slide (strict)"("Visible"=w318) -> ()  [unwired: 2 in, 2 out]
            n154 = Search and Replace String(input string=w319, search string="/Value  **", replace string="/Direction") -> (result string=w325:string)  [unwired: 5 in, 3 out]
            n155 = property on="Test Ring" class="Ring (strict)"("Visible"=w318) -> ()  [unwired: 2 in, 2 out]
            n156 = call <vilib>:"NT Read String.vi"("Name"=w325) -> ("String"=w323:string)  [unwired: 9 in, 1 out]
            n157 = Equal?(x="Both directions", y=w323) -> (x = y?=w321:bool)
            n158 = Not(x=w321) -> (.not. x?=w322:bool)
            n159 = property on="Rev/Fwd" class="Clust (strict)"("Visible"=w321) -> ()  [unwired: 2 in, 2 out]
            n160 = property on="On/Off" class="Bool (strict)"("Visible"=w322, "Caption.Text"=w320) -> ()  [unwired: 2 in, 2 out]
          }
          frame "Compressor", "Digital Out" {
            w328 = FALSE ("Visible")
            # "Get direction and finish"
            n161 = property on="Motor" class="Clust (strict)"("Visible"=w328) -> ()  [unwired: 2 in, 2 out]
            n162 = property on="Test Slider" class="Slide (strict)"("Visible"=w328) -> ()  [unwired: 2 in, 2 out]
            n163 = property on="Test Ring" class="Ring (strict)"("Visible"=w328) -> ()  [unwired: 2 in, 2 out]
            n164 = property on="On/Off" class="Bool (strict)"("Visible"=TRUE, "Caption.Text"=w329) -> ()  [unwired: 2 in, 2 out]
            n165 = property on="Rev/Fwd" class="Clust (strict)"("Visible"=FALSE) -> ()  [unwired: 2 in, 2 out]
          }
          frame "Camera" {
            n166 = call <vilib>:"Get Last Path Segment.vi"("String in"=w336) -> ("String out"=w337:string)  [unwired: 10 in]
            n167 = property on="On/Off" class="Bool (strict)"("Visible"=FALSE) -> ()  [unwired: 2 in, 2 out]
            n168 = property on="Motor" class="Clust (strict)"("Visible"=FALSE) -> ()  [unwired: 2 in, 2 out]
            n169 = property on="Rev/Fwd" class="Clust (strict)"("Visible"=FALSE) -> ()  [unwired: 2 in, 2 out]
            n170 = case shown="\"White Balance  **\"" w337 {
              tunnel: w336 -> [w343 w352 w361 w370 w379 _ w385]
              tunnel: w335 -> [w341 w349 w358 w367 w376 _ _]
              frame "Size  **" {
                n171 = Index Array(array=w341) -> (element=w340:cluster{string[]})  [unwired: 1 in]
                n172 = call <vilib>:"NT Read String.vi"("Name"=w343) -> ("String"=w342:string)  [unwired: 9 in, 1 out]
                n173 = Unbundle(w340) -> (w338:string[])
                n174 = Match First String(2:w338, 3:w342) -> (0:w339:i32)  [unwired: 1 out]
                n175 = property on="Test Ring" class="Ring (strict)"("Value"=w339, "Strings []"=w338) -> ()  [unwired: 2 in, 2 out]
                n176 = property on="Test Ring" class="Ring (strict)"("Visible"=TRUE) -> ()  [unwired: 2 in, 2 out]
                n177 = property on="Test Slider" class="Slide (strict)"("Visible"=FALSE) -> ()  [unwired: 2 in, 2 out]
              }
              frame "White Balance  **" {
                n178 = Index Array(array=w349, index=1) -> (element=w350:cluster{string[]})
                n179 = call <vilib>:"NT Read String.vi"("Name"=w352) -> ("String"=w351:string)  [unwired: 9 in, 1 out]
                n180 = Unbundle(w350) -> (w347:string[])
                n181 = Match First String(2:w347, 3:w351) -> (0:w346:i32)  [unwired: 1 out]
                n182 = property on="Test Ring" class="Ring (strict)"("Value"=w346, "Strings []"=w347) -> ()  [unwired: 2 in, 2 out]
                n183 = property on="Test Ring" class="Ring (strict)"("Visible"=TRUE) -> ()  [unwired: 2 in, 2 out]
                n184 = property on="Test Slider" class="Slide (strict)"("Visible"=FALSE) -> ()  [unwired: 2 in, 2 out]
              }
              frame "Exposure  **" {
                n185 = Index Array(array=w358, index=2) -> (element=w359:cluster{string[]})
                n186 = call <vilib>:"NT Read String.vi"("Name"=w361) -> ("String"=w360:string)  [unwired: 9 in, 1 out]
                n187 = Unbundle(w359) -> (w355:string[])
                n188 = Match First String(2:w355, 3:w360) -> (0:w356:i32)  [unwired: 1 out]
                n189 = property on="Test Ring" class="Ring (strict)"("Value"=w356, "Strings []"=w355) -> ()  [unwired: 2 in, 2 out]
                n190 = property on="Test Ring" class="Ring (strict)"("Visible"=TRUE) -> ()  [unwired: 2 in, 2 out]
                n191 = property on="Test Slider" class="Slide (strict)"("Visible"=FALSE) -> ()  [unwired: 2 in, 2 out]
              }
              frame "Exposure Priority  **" {
                n192 = Index Array(array=w367, index=3) -> (element=w368:cluster{string[]})
                n193 = call <vilib>:"NT Read String.vi"("Name"=w370) -> ("String"=w369:string)  [unwired: 9 in, 1 out]
                n194 = Unbundle(w368) -> (w364:string[])
                n195 = Match First String(2:w364, 3:w369) -> (0:w365:i32)  [unwired: 1 out]
                n196 = property on="Test Ring" class="Ring (strict)"("Value"=w365, "Strings []"=w364) -> ()  [unwired: 2 in, 2 out]
                n197 = property on="Test Ring" class="Ring (strict)"("Visible"=TRUE) -> ()  [unwired: 2 in, 2 out]
                n198 = property on="Test Slider" class="Slide (strict)"("Visible"=FALSE) -> ()  [unwired: 2 in, 2 out]
              }
              frame "Color Enable  **" {
                n199 = Index Array(array=w376, index=4) -> (element=w377:cluster{string[]})
                n200 = call <vilib>:"NT Read String.vi"("Name"=w379) -> ("String"=w378:string)  [unwired: 9 in, 1 out]
                n201 = Unbundle(w377) -> (w373:string[])
                n202 = Match First String(2:w373, 3:w378) -> (0:w374:i32)  [unwired: 1 out]
                n203 = property on="Test Ring" class="Ring (strict)"("Value"=w374, "Strings []"=w373) -> ()  [unwired: 2 in, 2 out]
                n204 = property on="Test Ring" class="Ring (strict)"("Visible"=TRUE) -> ()  [unwired: 2 in, 2 out]
                n205 = property on="Test Slider" class="Slide (strict)"("Visible"=FALSE) -> ()  [unwired: 2 in, 2 out]
              }
              frame Default {
                n206 = property on="Test Ring" class="Ring (strict)"("Visible"=FALSE) -> ()  [unwired: 2 in, 2 out]
                n207 = property on="Test Slider" class="Slide (strict)"("Visible"=FALSE) -> ()  [unwired: 2 in, 2 out]
              }
              frame "Brightness  **", "Color Level  **", "Compression  **", "FPS  **", "Sharpness  **" {
                n208 = call <vilib>:"NT Read Number.vi"("Name"=w385) -> ("Numeric"=w384:dbl)  [unwired: 9 in, 1 out]
                n209 = local write "Test Slider"(w384) -> ()
                n210 = property on="Test Slider" class="Slide (strict)"("Visible"=TRUE, "Scale.Maximum"=100.0 ("Scale.Range:Maximum")) -> ()  [unwired: 2 in, 2 out]
                n211 = property on="Test Ring" class="Ring (strict)"("Visible"=FALSE) -> ()  [unwired: 2 in, 2 out]
              }
            }
          }
        }
        n212 = property on="Progress" class="Clust (strict)"("Visible"=FALSE) -> ()  [unwired: 2 in, 2 out]
      }
      event "Test Name": Mouse Enter {
        # "Populate the ring with the list of tests"
        n213 = event-data() -> ()  [unwired: 1 in, 1 out]
        n214 = call <vilib>:"NT Read String Array.vi"("Name"="/TestMode/TestList") -> ("String Array"=w394:string[])  [unwired: 9 in, 1 out]
        n215 = Build Array (concatenate)("Select the test to run...", w394) -> (w393:string[])
        n216 = property on="Test Name" class="Ring (strict)"("Strings []"=w393) -> ()  [unwired: 2 in, 2 out]
      }
      event "Test Name": Value Change {
        w397 = FALSE ("Visible")
        # "Tell the robot the test name to run"
        n217 = event-data() -> ("NewVal"=w401:u16)  [unwired: 1 in]
        n218 = property on="Test Name" class="Ring (strict)"() -> ("Strings []"=w402:string[])  [unwired: 2 in, 2 out]
        n219 = local write "Progress"(T8 {"Test Progress"=0, "Test Progress Text"=""} ("Progress")) -> ()
        n220 = Index Array(array=w402, index=w401) -> (element=w400:string)
        n221 = call <vilib>:"NT Write String.vi"("String"=w400, "Name"="/TestMode/TestName") -> ()  [unwired: 9 in, 1 out]
        n222 = property on="Progress" class="Clust (strict)"("Visible"=TRUE) -> ()  [unwired: 2 in, 2 out]
        n223 = property on="Motor" class="Clust (strict)"("Visible"=w397) -> ()  [unwired: 2 in, 2 out]
        n224 = property on="Test Slider" class="Slide (strict)"("Visible"=w397) -> ()  [unwired: 2 in, 2 out]
        n225 = property on="On/Off" class="Bool (strict)"("Visible"=w397) -> ()  [unwired: 2 in, 2 out]
        n226 = property on="Rev/Fwd" class="Clust (strict)"("Visible"=w397) -> ()  [unwired: 2 in, 2 out]
        n227 = property on="Test Ring" class="Ring (strict)"("Visible"=w397) -> ()  [unwired: 2 in, 2 out]
      }
      event "Select Auto": Mouse Enter {
        # "Populate the combo box with the list of autonomous options"
        n228 = event-data() -> ()  [unwired: 1 in, 1 out]
        n229 = call <vilib>:"NT Read String Array.vi"("Name"="Auto List") -> ("String Array"=w404:string[])  [unwired: 9 in, 1 out]
        n230 = property on="Select Auto" class="CmbBox"("Strings[]"=w404) -> ()  [unwired: 2 in, 2 out]
      }
      event "Select Auto": Value Change {
        # "User modified the Auto Selection. Write to NT variable so robot knows."
        n231 = event-data() -> ("NewVal"=w408:string)  [unwired: 1 in]
        n232 = call <vilib>:"NT Write String.vi"("String"=w408, "Name"="Auto Selector") -> ()  [unwired: 9 in, 1 out]
      }
      event "Command Selection": Value Change {
        # "Get the params and show in table"
        n233 = event-data() -> ("NewVal"=w415:i32)  [unwired: 1 in]
        n234 = property on="Command Selection" class="MCListbox (strict)"() -> ("ItemNames"=w413:string[][])  [unwired: 2 in, 2 out]
        n235 = call <vilib>:"WPI_DashboardUpdate Command Params.vi"("NewVal"=w415, "Commands"=w413, "Param Tbl"=w414) -> ()  [unwired: 8 in, 1 out]
      }
      event "Execute Command": Value Change {
        # "Started one, Unique ID holds\nresponse"
        n236 = event-data() -> ()  [unwired: 1 in, 1 out]
        n237 = property on="Command Selection" class="MCListbox (strict)"() -> ("ItemNames"=w427:string[][])  [unwired: 2 in, 2 out]
        n238 = Index Array(array=w427, index (row)="Command Selection", index (col)=0) -> (element=w425:string)
        n239 = call <vilib>:"Invoke Commands.vi"("Command Params"="Command Params", "Function Name"=w425) -> ("Params"=w421:u8, "Started"=w420:bool)  [unwired: 7 in, 1 out]
        n240 = Array Subset(array="Command Params", length (row)=w421) -> (w422:string[][])  [unwired: 3 in]
        n241 = Select(t="Executing" ("Cmd Status"), s=w420, f="" ("Cmd Status")) -> (s? t:f=→"Cmd Status":string)
      }
      event "Command Selection": Double Click {
        n242 = event-data() -> ("Row"=w437:i32)  [unwired: 1 in]
        n243 = property on="Command Selection" class="MCListbox (strict)"() -> ("ItemNames"=w440:string[][])  [unwired: 2 in, 2 out]
        n244 = local read "Command Params"() -> (w435:string[][])
        n245 = Index Array(array=w440, index (row)=w437, index (col)=0) -> (element=w438:string)
        n246 = call <vilib>:"Invoke Commands.vi"("Command Params"=w435, "Function Name"=w438) -> ("Params"=w434:u8, "Started"=w429:bool)  [unwired: 7 in, 1 out]
        n247 = Array Subset(array=w435, length (row)=w434) -> (w433:string[][])  [unwired: 3 in]
        n248 = Select(t="Executing" ("Cmd Status"), s=w429, f="" ("Cmd Status")) -> (s? t:f=w430:string)
        n249 = local write "Cmd Status"(w430) -> ()
      }
      event "CheckList": Double Click {
        # "Shift clears all"
        # "Update symbols on the listbox"
        n250 = event-data() -> ("PlatMods.Shift"=w443:bool, "Row"=w445:i32)  [unwired: 1 in]
        n251 = case shown="True" w443 {
          tunnel: w445 -> [w449 _]
          tunnel: 1 -> [w448 _]
          frame False {
            n252 = property on="CheckList" class="LstBox (strict)"() -> ("Item Symbols"=w447:i32[])  [unwired: 2 in, 2 out]
            n253 = Replace Array Subset(array=w447, new element=w448, index=w449) -> (w446:i32[])
            n254 = property on="CheckList" class="LstBox (strict)"("Item Symbols"=w446) -> ()  [unwired: 2 in, 2 out]
          }
          frame True {
            w450 = 0 ("Top Row")
            n255 = property on="CheckList" class="LstBox (strict)"() -> ("Number of Rows"=w452:u32)  [unwired: 2 in, 2 out]
            n256 = Initialize Array(0, w452) -> (w451:i32[])
            n257 = property on="CheckList" class="LstBox (strict)"("Top Row"=w450, "Value"=w450, "Item Symbols"=w451) -> ()  [unwired: 2 in, 2 out]
          }
        }
      }
      event "CheckList": Key Down {
        # "Update symbols on the listbox\nLeft and right keys check and uncheck"
        n258 = event-data() -> ("VKey"=w457:T22)  [unwired: 1 in]
        n259 = case shown="\"Left\", \"Right\"" w457 {
          selector: w457 -> [w462 _]
          tunnel: eventvkey."Left" ("VKey") -> [w460 _]
          frame "Left", "Right" {
            n260 = Equal?(x=w460, y=w462) -> (x = y?=w461:bool)
            n261 = Select(t=0, s=w461, f=1) -> (s? t:f=w463:i32)
            n262 = property on="CheckList" class="LstBox (strict)"() -> ("Item Symbols"=w466:i32[])  [unwired: 2 in, 2 out]
            n263 = Replace Array Subset(array=w466, new element=w463, index="CheckList") -> (w465:i32[])
            n264 = property on="CheckList" class="LstBox (strict)"("Item Symbols"=w465) -> ()  [unwired: 2 in, 2 out]
          }
          frame Default {
          }
        }
      }
      event "DB Camera Config": Value Change {
        # "Show or hide the cluster of controls, store in ini file"
        n265 = event-data() -> ("NewVal"=w471:bool)  [unwired: 1 in]
        n266 = case shown="False" w471 {
          tunnel: w470 -> [w480 _]
          tunnel: [w473 w491] -> w469
          tunnel: w468 -> [w472 w491]
          frame False {
            w487 = "Camera"
            w490 = FALSE ("Visible")
            n267 = local read "Camera Settings"() -> (w479:T2)
            n268 = Index Array(array=w480) -> (element=w483:cluster{string[]})  [unwired: 1 in]
            n269 = Unbundle(w479) -> ("Frame Rate"=w478:i32, "Compression"=w477:i32, "Size"=w481:u16)
            n270 = Unbundle(w483) -> (w482:string[])
            n271 = Index Array(array=w482, index=w481) -> (element=w476:string)
            n272 = call-poly <vilib>:"Write Key.vi"("section"=w487, "value"=w476, "key"="Size", "refnum"=w472) -> ("refnum out"=w489:T20)  [unwired: 2 in, 5 out]
            n273 = call-poly <vilib>:"Write Key.vi"("section"=w487, "value"=w478, "key"="FrameRate", "refnum"=w489) -> ("refnum out"=w488:T20)  [unwired: 1 in, 6 out]
            n274 = property on="Camera Settings" class="Clust (strict)"("Visible"=w490) -> ()  [unwired: 2 in, 2 out]
            n275 = local write "DB Camera Config"(w490) -> ()
            n276 = call-poly <vilib>:"Write Key.vi"("section"=w487, "value"=w477, "key"="Compression", "refnum"=w488) -> ("refnum out"=w474:T20)  [unwired: 1 in, 6 out]
            n277 = call <vilib>:"Close Config Data.vi"("refnum"=w474) -> ("file path"=w475:path)  [unwired: 2 in, 8 out]
            n278 = call <vilib>:"Open Config Data.vi"("configuration file path"=w475) -> ("refnum"=w473:T20)  [unwired: 8 in, 2 out]
          }
          frame True {
            n279 = property on="Camera Settings" class="Clust (strict)"("Visible"=TRUE) -> ()  [unwired: 2 in, 2 out]
          }
        }
      }
      event "Camera Settings": Value Change {
        # "Update summary string when any elements of DB camera change"
        n280 = event-data() -> ("NewVal"=w505:T2)  [unwired: 1 in]
        n281 = Index Array(array=w501) -> (element=w500:cluster{string[]})  [unwired: 1 in]
        n282 = Unbundle(w505) -> ("Frame Rate"=w496:i32, "Compression"=w495:i32, "Size"=w498:u16)
        n283 = Unbundle(w500) -> (w499:string[])
        n284 = Index Array(array=w499, index=w498) -> (element=w497:string)
        n285 = Format Into String(format string="%s   %dfps   %d%%", w497, w496, w495) -> (resulting string=w502:string)  [unwired: 2 in, 1 out]
        n286 = Build Array(w502) -> (w503:string[])
        n287 = property on="DB Camera Config" class="Bool (strict)"("Strings [4]"=w503) -> ()  [unwired: 2 in, 2 out]
      }
      event "Motor.Enable": Value Change {
        # "When the test mode otor enable helper is set, update that\ntree row item's value"
        n288 = event-data() -> ("NewVal"=w512:bool)  [unwired: 1 in]
        n289 = Unbundle("Motor") -> ("Value"=w511:dbl)  [unwired: 1 out]
        n290 = Select(t=w511, s=w512, f=0.0) -> (s? t:f=w509:dbl)
        n291 = call <vilib>:"NT Write Number.vi"("Numeric"=w509, "Name"=w508) -> ()  [unwired: 9 in, 1 out]
      }
      event "Test Slider": Value Change {
        # "When the test mode slider helper is set, update that\ntree row item's value"
        n292 = event-data() -> ("NewVal"=w516:dbl)  [unwired: 1 in]
        n293 = call <vilib>:"NT Write Number.vi"("Numeric"=w516, "Name"=w517) -> ()  [unwired: 9 in, 1 out]
      }
      event "On/Off": Value Change {
        # "When the test mode on/off helper value is set, update that\ntree row item's value"
        n294 = event-data() -> ("NewVal"=w522:bool)  [unwired: 1 in]
        n295 = Boolean To (0,1)(Boolean=w522) -> (0, 1=w521:i16)
        n296 = call <vilib>:"NT Write Number.vi"("Numeric"=w521, "Name"=w520) -> ()  [unwired: 9 in, 1 out]
      }
      event "Rev/Fwd": Value Change {
        # "When the test mode helper value for relays is set, update that\ntree row item's value"
        n297 = event-data() -> ("NewVal.Forward"=w531:bool, "NewVal.Reverse"=w530:bool)  [unwired: 1 in]
        n298 = Boolean To (0,1)(Boolean=w531) -> (0, 1=w527:i16)
        n299 = Boolean To (0,1)(Boolean=w530) -> (0, 1=w529:i16)
        n300 = Negate(x=w529) -> (-x=w528:i16)
        n301 = Add(x=w527, y=w528) -> (x+y=w526:i16)
        n302 = call <vilib>:"NT Write Number.vi"("Numeric"=w526, "Name"=w525) -> ()  [unwired: 9 in, 1 out]
      }
      event "Test Ring": Value Change {
        # "When a test mode helper value is selected from the ring,\nset the tree item's variable to the string value"
        n303 = event-data() -> ("NewVal"=w536:u16)  [unwired: 1 in]
        n304 = property on="Test Ring" class="Ring (strict)"() -> ("Strings []"=w537:string[])  [unwired: 2 in, 2 out]
        n305 = Index Array(array=w537, index=w536) -> (element=w535:string)
        n306 = call <vilib>:"NT Write String.vi"("String"=w535, "Name"=w534) -> ()  [unwired: 9 in, 1 out]
      }
      event "Rec Mode": Value Change {
        # "Update globals for recording mode and path to read log from.\nClear when logging and let NetworkTables set path for vision to\nuse."
        n307 = event-data() -> ("NewVal"=w549:enum32{"Stop", "Record", "Playback"})  [unwired: 1 in]
        n308 = global write "WPI_DashboardLogging Global.vi" "Logging Filename"(path "") -> ()
        n309 = global write "WPI_DashboardLogging Global.vi" "Recording"(w549) -> ()
        n310 = case shown="\"Playback\"" w549 {
          tunnel: w548 -> [_ w551 w560]
          tunnel: [_ _ w559] -> w545
          tunnel: [_ _ w558] -> _
          tunnel: w543 -> [_ _ w556]
          tunnel: cluster{i32, i32} {-250, 170} -> [_ _ w555]
          tunnel: [_ _ T23 {"Image Size"=TRUE, "Image Type"=TRUE, "Pixel Value"=TRUE, "ROI Information"=TRUE, "Zoom Factor"=FALSE} ("Image Information Shown:All Elements")] -> w541
          tunnel: [_ _ TRUE ("Zoom Factor")] -> w540
          tunnel: w539 -> [_ _ w552]
          frame Default {
          }
          frame "Stop", "Record" {
            # "Place Window too"
            n311 = invoke class="VI" method="FP.Close"(reference=w551) -> (reference out=w550:refnum<vi>)  [unwired: 2 in, 2 out]
            n312 = invoke class="VI" method="Abort VI"(reference=w550) -> ()  [unwired: 2 in, 3 out]
          }
          frame "Playback" {
            n313 = call "Open Playback Panel.vi"("Offset"=w555, "DB VI Ref"=w556, "Playback in"=w560) -> ("Playback out"=w557:refnum<vi>)  [unwired: 8 in]
            n314 = register-events(w557, w552) -> (reference out=w559:refnum<event-registration>, error out=w558:errorcluster)  [unwired: 2 in]
          }
        }
        n315 = property on="Camera Image" class="ImageControl"("Image Information Shown"=w541, "Image Information Visible"=w540) -> ()  [unwired: 2 in, 2 out]
        n316 = call <vilib>:"WPI_DashboardNT Log FieldName Cache.vi"("Operation"=enum16{"Lookup/Add", "Index", "Clear"}."Clear") -> ()  [unwired: 8 in, 3 out]
      }
      event Panel Close {
        w562 = enum32{"Stop", "Record", "Playback"}."Stop" ("Rec Mode")
        # "Playback window has been closed, abort"
        n317 = event-data() -> ()  [unwired: 1 in, 4 out]
        n318 = local write "Rec Mode"(w562) -> ()
        n319 = global write "WPI_DashboardLogging Global.vi" "Recording"(w562) -> ()
      }
      event Panel Close {
        # "Abort playback window and ourself"
        n320 = event-data() -> ()  [unwired: 1 in, 4 out]
        n321 = invoke class="VI" method="FP.Close"(reference=w568) -> (reference out=w567:refnum<vi>)  [unwired: 2 in, 2 out]
        n322 = invoke class="VI" method="Abort VI"(reference=w567) -> (error out=w566:errorcluster)  [unwired: 2 in, 2 out]
        n323 = invoke class="VI" method="Abort VI"(error in=w566) -> ()  [unwired: 2 in, 3 out]
      }
      event User Event {
        n324 = event-data() -> ("IDs"=w576:cluster{"RPC field ID":u16, "Unique ID":u16}, "String"=w575:string)  [unwired: 1 in]
        n325 = Bundle("IDs"=w576, "String"=w575) -> (w574:T9)  [unwired: 1 in]
        n326 = call <vilib>:"Retrieve RPC Response.vi"("RPC Response"=w574) -> ("Output"=w571:string[][])  [unwired: 10 in]
        n327 = Build Array (concatenate)(w569, w571) -> (w570:string[][])
        n328 = local write "Command Params"(w570) -> ()
        n329 = local write "Cmd Status"("" ("Cmd Status")) -> ()
      }
      event "Vision": Value Change {
        # "Enable/Disable Compression slider.\nHW USB is hard-coded into the camera"
        n330 = event-data() -> ("NewVal"=w583:u16)  [unwired: 1 in]
        n331 = Equal?(x=w583, y=u32 2 ("milliseconds to wait")) -> (x = y?=w581:bool)
        n332 = Select(t=T24."Disabled and Grayed Out" ("Disabled"), s=w581, f=T24."Enabled" ("Disabled")) -> (s? t:f=w578:T24)
        n333 = property on="Compression" class="Slide (strict)"("DisabledEnum"=w578) -> ()  [unwired: 2 in, 2 out]
      }
      event "Tree": Double Click {
        n334 = event-data() -> ("PlatMods"=w588:T27, "Tag"=w587:string)  [unwired: 1 in]
        n335 = Unbundle(w588) -> ("Shift"=w586:bool)  [unwired: 4 out]
        n336 = Not(x=w586) -> (.not. x?=w585:bool)
        n337 = call <vilib>:"NT Update Persistence.vi"("Persistence"=w585, "Name"=w587) -> ()  [unwired: 9 in, 1 out]
      }
    }
  }
  n338 = while {
    tunnel: w47 -> [w592]
    i -> [w595]
    stop <- FALSE stop-if-true
    n339 = Wait (ms)(milliseconds to wait=u32 100) -> ()  [unwired: 1 out]
    n340 = case shown="\"Playback\"" "Rec Mode" {
      tunnel: w595 -> [_ _ w610]
      tunnel: [u32 2829099 ("Base Color") u32 11141120 ("Target Color") w599] -> w591
      frame "Stop", Default {
        # "Reset the color, extra updates don't cost much"
      }
      frame "Record" {
      }
      frame "Playback" {
        # "Playback"
        n341 = Quotient & Remainder(x=w610, y=u32 50 ("milliseconds to wait")) -> (x-y*floor(x/y)=w606:u32)  [unwired: 1 out]
        n342 = Divide(x=w606, y=u32 50 ("milliseconds to wait")) -> (x/y=w603:dbl)
        n343 = Multiply(x=6.283185307179586, y=w603) -> (x*y=w608:dbl)
        n344 = Sine(x=w608) -> (sin(x)=w607:dbl)
        n345 = Absolute Value(x=w607) -> (abs(x)=w600:dbl)
        n346 = call "Interpolate RGB Color.vi"("Proportion"=w600, "Target Color"=u32 30976, "Base Color"=u32 2829099) -> ("Result Color"=w599:u32)  [unwired: 8 in]
      }
    }
    n347 = property class="Pane"(reference=w592, "PaneColor"=w591) -> ()  [unwired: 1 in, 2 out]
  }
  n348 = local write "Dashboard Tab"(T1."Drive" ("Dashboard Tab")) -> ()
  n349 = property on="On/Off" class="Bool (strict)"("Visible"=w15) -> ()  [unwired: 2 in, 2 out]
  n350 = property on="Motor" class="Clust (strict)"("Visible"=w15) -> ()  [unwired: 2 in, 2 out]
  n351 = property on="Progress" class="Clust (strict)"("Visible"=w15) -> ()  [unwired: 2 in, 2 out]
  n352 = property on="Test Ring" class="Ring (strict)"("Visible"=w15) -> ()  [unwired: 2 in, 2 out]
  n353 = property on="Rev/Fwd" class="Clust (strict)"("Visible"=w15) -> ()  [unwired: 2 in, 2 out]
  n354 = property on="Camera Settings" class="Clust (strict)"("Visible"=w15) -> ()  [unwired: 2 in, 2 out]
  n355 = while {
    tunnel: u16 1741 ("timeout ms (25000)") -> [w612]
    stop <- FALSE stop-if-true
    n356 = TCP Create Listener(10:w612) -> (0:w611:errorcluster, 3:w613:refnum<k5>)  [unwired: 4 in, 1 out]
    n357 = case shown="No Error" w611 {
      selector: w611 -> [w615 _]
      tunnel: w613 -> [w616 _]
      frame No Error {
        n358 = while {
          tunnel: w616 -> [w619]
          tunnel: w615 -> [w618]
          stop <- FALSE stop-if-true
          n359 = TCP Wait On Listener(8:w618, 11:w619) -> (0:w620:errorcluster, 4:w621:refnum<k5>)  [unwired: 2 in, 3 out]
          n360 = local write "TCP"(w621) -> ()
          n361 = case shown="No Error" w620 {
            frame No Error {
            }
            frame Error {
              n362 = Wait (ms)(milliseconds to wait=u32 1000) -> ()  [unwired: 1 out]
            }
          }
        }
      }
      frame Error {
        n363 = Wait (ms)(milliseconds to wait=u32 1000) -> ()  [unwired: 1 out]
      }
    }
  }
  n364 = local write "DB Camera Config"(w15) -> ()
  n365 = local write "Command Params"(string[][] [] ("Command Params")) -> ()
  n366 = global write "WPI_DashboardLogging Global.vi" "Recording"(w41) -> ()
  n367 = local write "Command Selection"(u16 0 ("milliseconds to wait")) -> ()
  n368 = local write "Rec Mode"(w41) -> ()
  n369 = while {
    stop <- FALSE stop-if-true
    n370 = call "Vision Acquisition"() -> ("Image Out"=→"Image Out":T7)  [unwired: 25 in, 2 out]
  }
